vi "AddI32.vi"(4 "y":i32, 5 "x":i32) -> (1 "x+y":i32, 2 "Overflow?":bool)   [LabVIEW 2017, in "GPOverflow.lvlib"]
doc: "Adds <B>x</B> to <B>y</B> keeping track of numeric overflow.\n\n<B>Overflow?</B> will be True if positive or negative overflow occurred. The output will saturate in case of overflow.\n\nThis VI is inlined.\n\nSteen Schmidt\nGPower\n8/8 2013"
uses:
  GPOverflow.lvlib
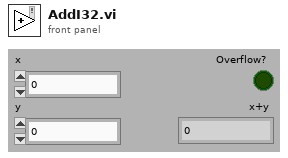
[diagram p1: front panel]
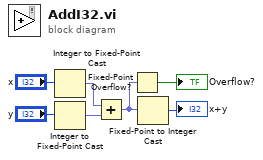
[diagram p0: block diagram]
diagram:
  n1 = Integer to Fixed-Point Cast(integer="x") -> (fixed-point=w5:fxp<+/-,32,32>)  [unwired: 1 in]
  n2 = Integer to Fixed-Point Cast(integer="y") -> (fixed-point=w4:fxp<+/-,32,32>)  [unwired: 1 in]
  n3 = Add(x=w5, y=w4) -> (x+y=w3:fxp<+/-,32,32>)
  n4 = Fixed-Point Overflow?(1:w3) -> (0:→"Overflow?":bool)
  n5 = Fixed-Point to Integer Cast(1:w3) -> (0:→"x+y":i32)
